vi "Threshold (Binary).vi"(4 "Max Value (Default: 255)":u8=255, 6 "Invert? (Default: False)":bool, 7 "Threshold":u8, 8 "error in (no error)":errorcluster, 10 "Threshold Result in":T1, 11 "Greyscale Image-Source in":T1) -> (0 "error out":errorcluster, 3 "Threshold Result":T1)   [LabVIEW 2020, in "image.lvlib"]
doc: "Convert the Greyscale Image into a Binary Image by applying an adaptive threshold."
uses:
  image.lvlib
  Greyscale Image.ctl
  ThresholdTypes.ctl
  <vilib>/Utility/error.llb/Error Cluster From Error Code.vi
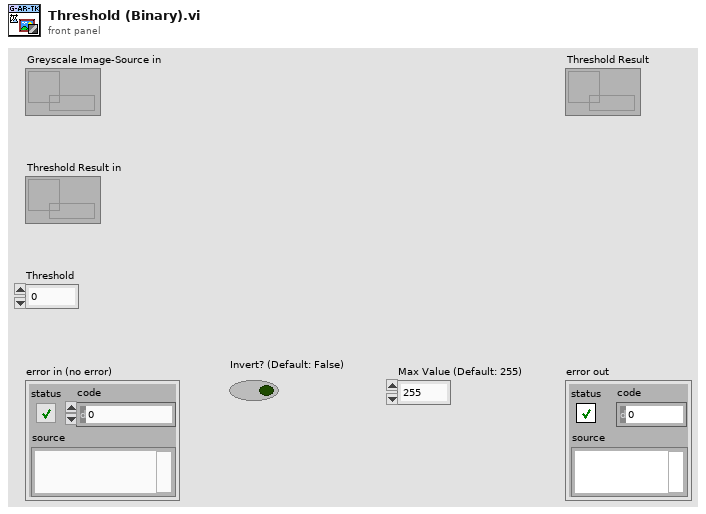
[diagram p1: front panel]
types:
  T1 = typedef "image.lvlib/Greyscale Image.ctl" = refnum<data-value>
  T2 = typedef "image.lvlib/ThresholdTypes.ctl" = enum8{"THRESH_BINARY", "THRESH_BINARY_INV", "THRESH_TRUNC", "THRESH_TOZERO", "THRESH_TOZERO_INV", "THRESH_MASK", "THRESH_OTSU", "THRESH_TRIANGLE"}
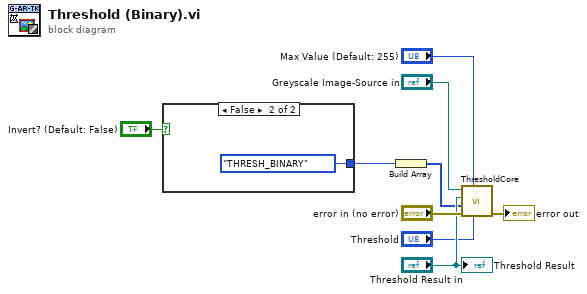
[diagram p0: block diagram]
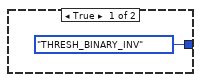
[diagram p2: hidden frame]
diagram:
  n1 = case shown="False" "Invert? (Default: False)" {
    tunnel: [ThresholdTypes."THRESH_BINARY_INV" ("Threshold Types") ThresholdTypes."THRESH_BINARY" ("Threshold Types")] -> w2
    frame True {
    }
    frame False {
    }
  }
  n2 = Build Array(w2) -> (w1:T2[])
  n3 = call "ThresholdCore.vi"("Threshold"="Threshold", "Max Value"="Max Value (Default: 255)", "error in (no error)"="error in (no error)", "Mode"=w1, "Threshold Result in"="Threshold Result in", "Greyscale Image-Source in"="Greyscale Image-Source in") -> ("error out"=→"error out":errorcluster)  [unwired: 5 in]
  "Threshold Result" <- "Threshold Result in"
